vi "PAN_ExtractCmdID.vi"(10 "command in":string) -> (1 "cmdID":string, 2 "cmd out":string)   [LabVIEW 2016]
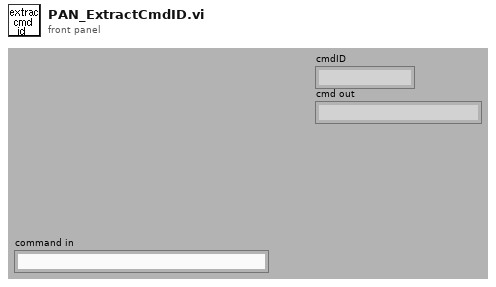
[diagram p1: front panel]
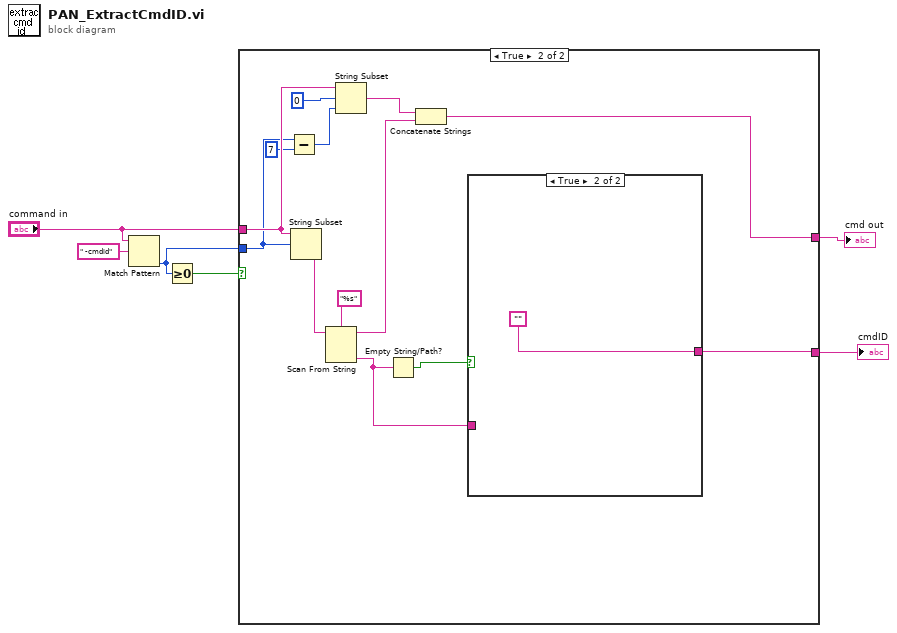
[diagram p0: block diagram]
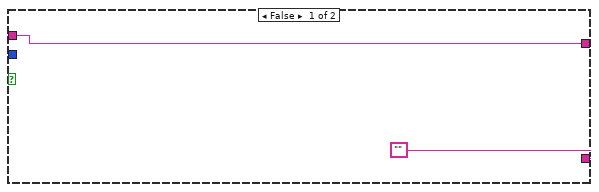
[diagram p2: hidden frame]
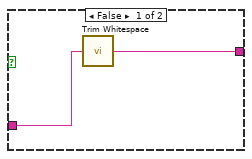
[diagram p3: hidden frame]
diagram:
  n1 = Match Pattern(string="command in", regular expression=" -cmdid") -> (offset past match=w1:i32)  [unwired: 4 out]
  n2 = Greater Or Equal To 0?(x=w1) -> (x >= 0?=w4:bool)
  n3 = case shown="True" w4 {
    tunnel: ["" w21] -> w5
    tunnel: w1 -> [_ w11]
    tunnel: "command in" -> [w7 w17]
    tunnel: [w7 w14] -> w2
    frame False {
    }
    frame True {
      n4 = Subtract(x=w11, y=7) -> (x-y=w9:i32)
      n5 = String Subset(string=w17, offset (0)=w11) -> (substring=w20:string)  [unwired: 1 out]
      n6 = Scan From String(format string="%s", input string=w20) -> (remaining string=w15:string, output 1=w13:string)  [unwired: 2 in, 3 out]
      n7 = String Subset(string=w17, offset (0)=0, length (rest)=w9) -> (substring=w16:string)
      n8 = Empty String/Path?(string/path=w13) -> (empty?=w18:bool)
      n9 = Concatenate Strings(w16, w15) -> (w14:string)
      n10 = case shown="True" w18 {
        tunnel: [w22 ""] -> w21
        tunnel: w13 -> [w23 _]
        frame False {
          n11 = call <vilib>:"Trim Whitespace.vi"("string"=w23) -> ("trimmed string"=w22:string)  [unwired: 1 in]
        }
        frame True {
        }
      }
    }
  }
  "cmdID" <- w5
  "cmd out" <- w2
